vi "ReadBinaryFromDisk.vi"(3 "size to read (count)":i64, 4 "offset (in bytes) (0)":i64, 5 "Set Position?":bool, 6 "Read or Write Path":path) -> (1 "data (U8)":u8[](array[numeric]), 2 "refnum out":refnum<file>)   [LabVIEW 2014]
panel:
  out "data (I16)":i16[](array[numeric])
  in  "Data type":enum16{"U8", "I16"}(ring)
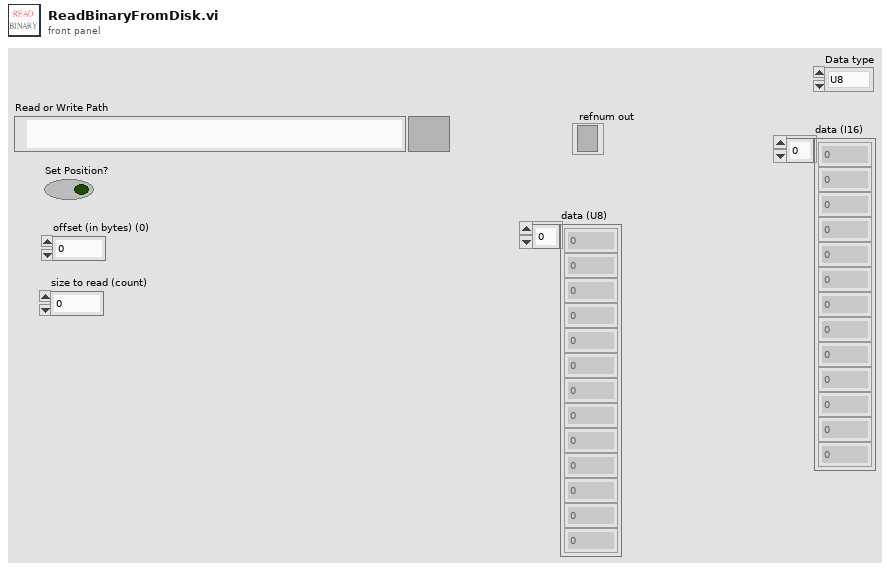
[diagram p1: front panel]
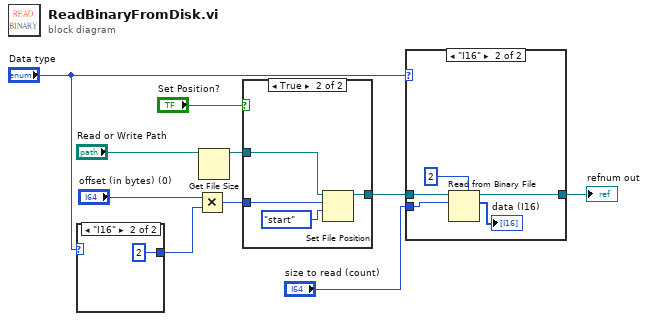
[diagram p0: block diagram]
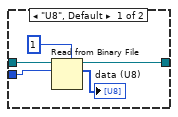
[diagram p3: hidden frame]
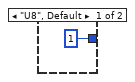
[diagram p4: hidden frame]
diagram:
  n1 = case shown="\"I16\"" "Data type" {
    tunnel: [u8 1 i16 2] -> w2
    frame "U8", Default {
    }
    frame "I16" {
    }
  }
  n2 = Multiply(x="offset (in bytes) (0)", y=w2) -> (x*y=w1:i64)
  n3 = Get File Size(file="Read or Write Path") -> (refnum out=w7:refnum<file>)  [unwired: 1 in, 2 out]
  n4 = case shown="True" "Set Position?" {
    tunnel: w7 -> [w13 w17]
    tunnel: w1 -> [_ w16]
    tunnel: [w13 w14] -> w6
    frame False {
    }
    frame True {
      n5 = Set File Position(offset (in bytes) (0)=w16, refnum=w17, from (0:start)=enum16{"start", "end", "current"}."start") -> (refnum out=w14:refnum<file>)  [unwired: 1 in, 1 out]
    }
  }
  n6 = case shown="\"I16\"" "Data type" {
    tunnel: "size to read (count)" -> [w20 w26]
    tunnel: w6 -> [w21 w25]
    tunnel: [w18 w23] -> w4
    frame "U8", Default {
      n7 = Read from Binary File(5:u8 1, 10:w20, 11:w21) -> (2:→"data (U8)":u8[], 3:w18:refnum<file>)  [unwired: 3 in, 2 out]
    }
    frame "I16" {
      n8 = Read from Binary File(5:i16 2, 10:w26, 11:w25) -> (2:→"data (I16)":i16[], 3:w23:refnum<file>)  [unwired: 3 in, 2 out]
    }
  }
  "refnum out" <- w4
